vi "Day 7 Tasks Shift Registers.vi"() -> ()   [LabVIEW 2026]
panel:
  out "Array 2":i32[](array[numeric])
  out "Array":dbl[](array[numeric])
  out "OUTPUT SUM":i32
  in  "stop":bool
  # "DAY 7 - TASK 1"
  # "DAY 7 - TASK 2"
  # "DAY 7 - TASK 2"
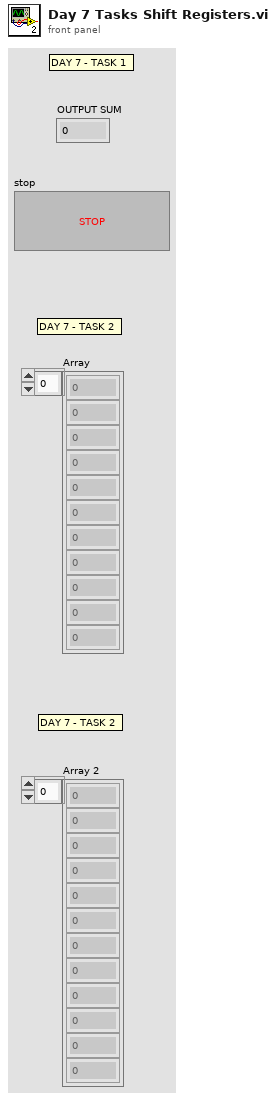
[diagram p1: front panel]
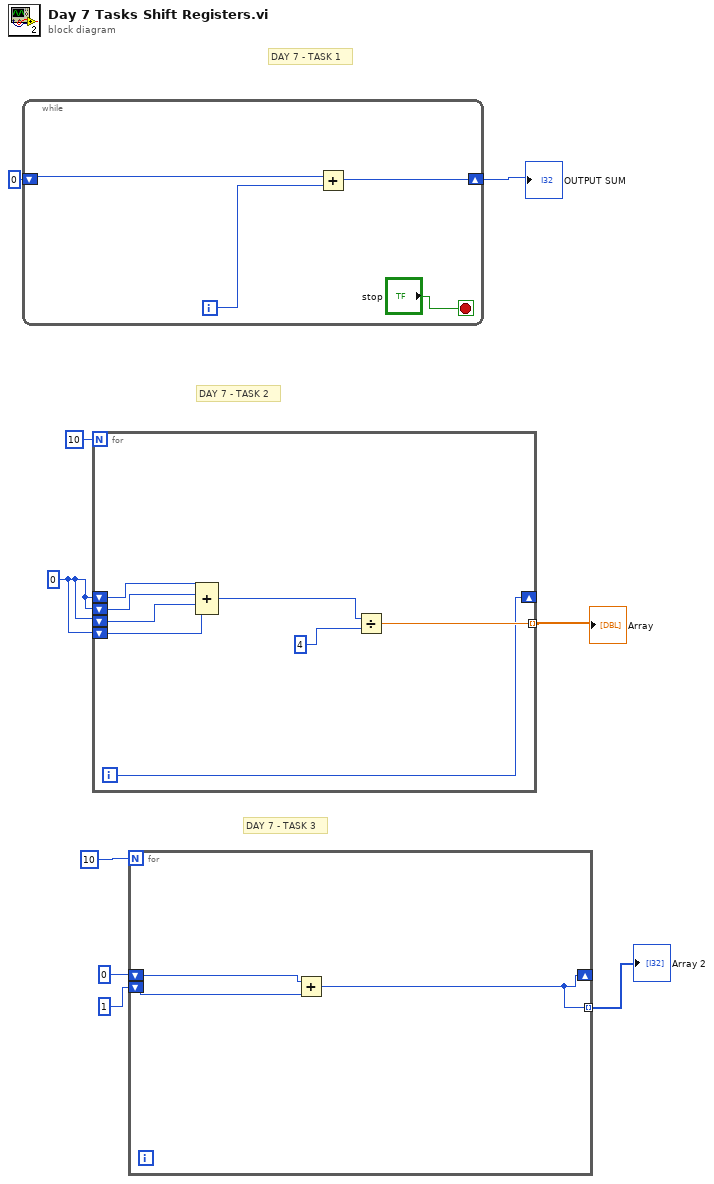
[diagram p0: block diagram]
diagram:
  w5 = 0
  # "DAY 7 - TASK 3"
  # "DAY 7 - TASK 2"
  # "DAY 7 - TASK 1"
  n1 = while {
    shift-right: [w11] -> w8
    shift-left: 0 -> [w12]
    i -> [w13]
    stop <- "stop" stop-if-true
    n2 = Add(x=w12, y=w13) -> (x+y=w11:i32)
  }
  "OUTPUT SUM" <- w8
  n3 = for {
    N: 10 -> [_]
    shift-right: [w14] -> _
    shift-left: w5 -> [w19]
    tunnel: [w20] -> w6 mode=indexing
    shift-left: w5 -> [w18]
    shift-left: w5 -> [w17]
    shift-left: w5 -> [w16]
    i -> [w14]
    n4 = Compound Arithmetic op=ADD(w19, w18, w17, w16) -> (w15:i32)
    n5 = Divide(x=w15, y=4) -> (x/y=w20:dbl)
  }
  "Array" <- w6
  n6 = for {
    N: 10 -> [_]
    shift-right: [w22] -> _
    shift-left: 0 -> [w24]
    shift-left: 1 -> [w23]
    tunnel: [w22] -> w2 mode=indexing
    n7 = Add(x=w24, y=w23) -> (x+y=w22:i32)
  }
  "Array 2" <- w2
